vi "Main.vi"() -> ()   [LabVIEW 2014]
panel:
  out "error out":errorcluster
  in  "Stop Button":bool
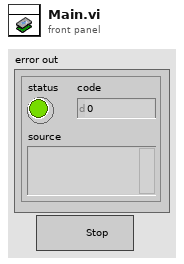
[diagram p1: front panel]
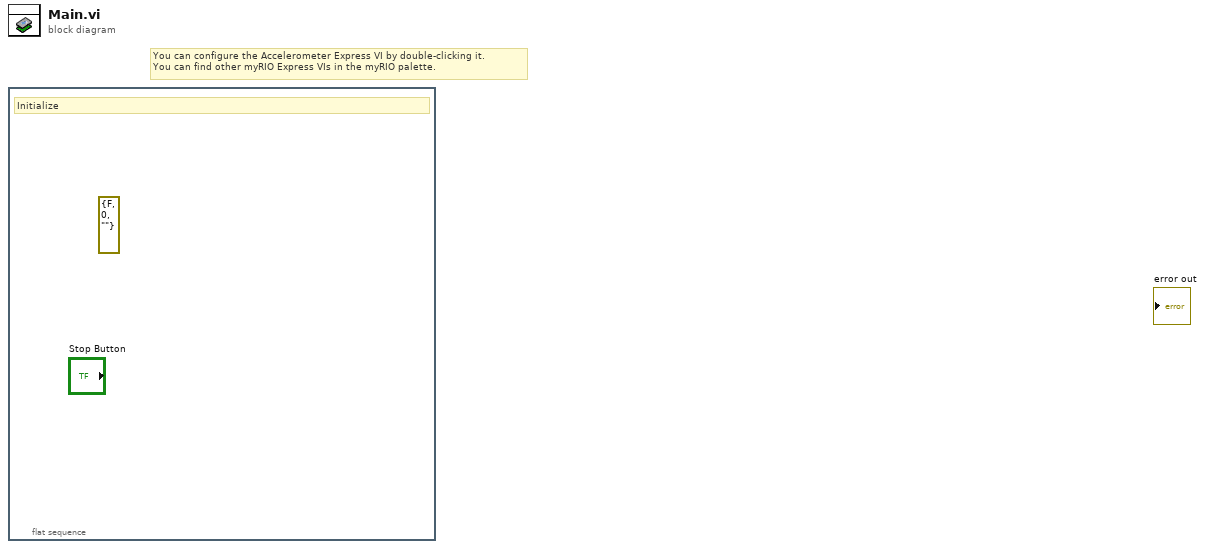
[diagram p0: block diagram]
diagram:
  # "You can configure the Accelerometer Express VI by double-clicking it.\nYou can find other myRIO Express VIs in the myRIO palette."
  n1 = flat-sequence {
    frame #0 {
      w1 = errorcluster {"status"=FALSE, "code"=0, "source"=""} ("error out")
      # "Initialize"
    }
  }
